vi "Update Screen - All.vi"(8 "error in (no error)":errorcluster, 11 "Update Screen":T1) -> (0 "error out":errorcluster)   [LabVIEW 2016]
uses:
  Update Screen.ctl
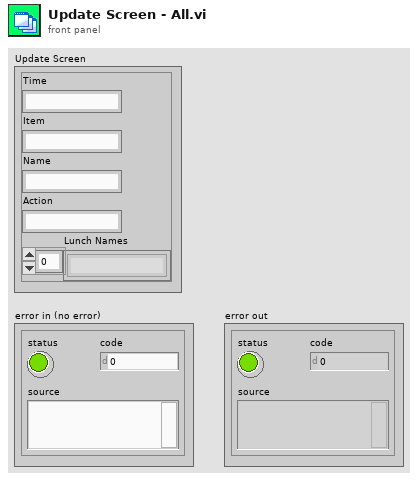
[diagram p1: front panel]
types:
  T1 = typedef "Update Screen.ctl" = cluster{"Time":string, "Item":string, "Name":string, "Action":string, "Lunch Names":string[]}
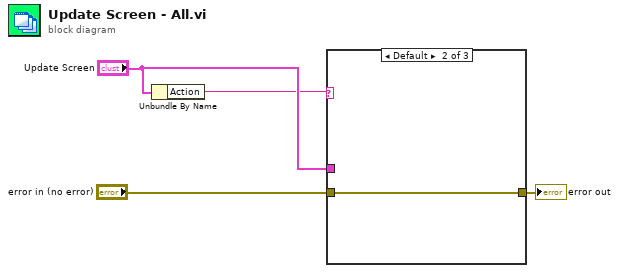
[diagram p0: block diagram]
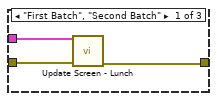
[diagram p2: hidden frame]
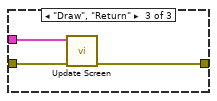
[diagram p3: hidden frame]
diagram:
  n1 = Unbundle By Name("Update Screen") -> ("Action"=w1:string)
  n2 = case shown="Default" w1 {
    tunnel: [w6 w8 w11] -> w4
    tunnel: "error in (no error)" -> [w7 w8 w10]
    tunnel: "Update Screen" -> [w5 _ w9]
    frame "First Batch", "Second Batch" {
      n3 = call "Update Screen - Lunch.vi"("error in (no error)"=w7, "Update Screen"=w5) -> ("error out"=w6:errorcluster)  [unwired: 9 in]
    }
    frame Default {
    }
    frame "Draw", "Return" {
      n4 = call "Update Screen.vi"("error in (no error)"=w10, "Update Screen"=w9) -> ("error out"=w11:errorcluster)  [unwired: 9 in]
    }
  }
  "error out" <- w4
